vi "ReadFlat.vi"() -> (3 "Flat_mirror":i32[](array[numeric]))   [LabVIEW 2011]
uses:
  <vilib>/Utility/file.llb/Read From Spreadsheet File (string).vi
panel:
  out "output 2":string
  out "output 1":string
  out "output 3":i32
  out "element":string
  out "all rows":string[][](array[string])
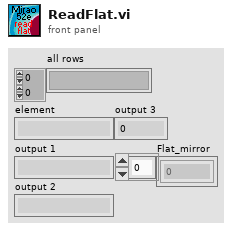
[diagram p1: front panel]
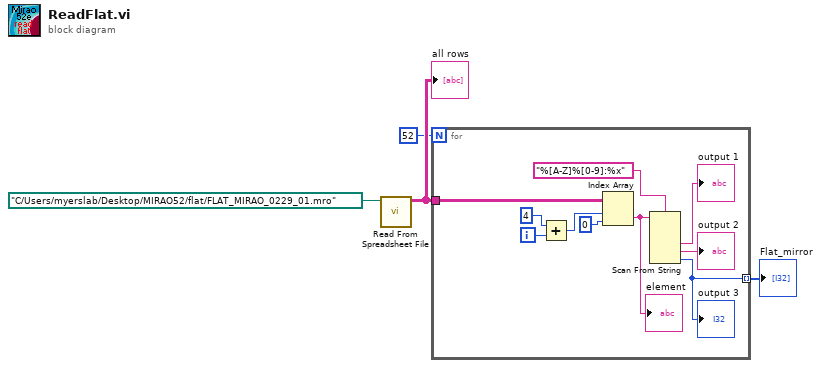
[diagram p0: block diagram]
diagram:
  n1 = call-poly <vilib>:"Read From Spreadsheet File.vi"("file path (dialog if empty)"=path "C:/Users/myerslab/Desktop/MIRAO52/flat/FLAT_MIRAO_0229_01.mro") -> ("all rows"=w4:string[][])  [unwired: 6 in, 4 out]
  "all rows" <- w4
  n2 = for {
    N: 52 -> [_]
    tunnel: w4 -> [w12]
    tunnel: [w5] -> w1 mode=indexing
    i -> [w14]
    n3 = Add(x=4, y=w14) -> (x+y=w11:i32)
    n4 = Index Array(array=w12, index (row)=w11, index (col)=0 ("disabled index (col)")) -> (element=w9:string)
    "element" <- w9
    n5 = Scan From String(format string="%[A-Z]%[0-9]:%x", input string=w9) -> (output 1=→"output 1":string, output 2=→"output 2":string, output 3=w5:i32)  [unwired: 5 in, 3 out]
    "output 3" <- w5
  }
  "Flat_mirror" <- w1
